vi "SIRDualSlices.vi"(8 "P":cluster{"x":dbl, "y":dbl, "z":dbl}={"x"=1.0, "y"=-5.0, "z"=1.0} {"x" format="%.2f"; "z" format="%.2f"; "y" format="%.2f"}, 9 "Variables":T2={"sound spd (cm/s)"=150000, "time step (s)"=1e-09} {"time step (s)" format="%.2e"}, 11 "strip":cluster{"Radius":dbl, "h":dbl, "a":dbl}={"Radius"=10.0, "h"=3.0, "a"=5.0} {"Radius" format="%.2f"; "a" format="%.2f"; "h" format="%.2f"}) -> (0 "r values":T1 {"r5" format="%.4f"; "r4" format="%.4f"; "r3" format="%.4f"; "r2" format="%.4f"; "r1" format="%.4f"; "r0" format="%.4f"}, 1 "lower":dbl[](graph), 2 "upper":dbl[](graph), 3 "h outer strips":dbl[](graph), 4 "delay out":i32, 5 "cap delay pts":i32, 7 "h cap":dbl[](array[numeric]) format="%.2f")   [LabVIEW 2022 SP3]
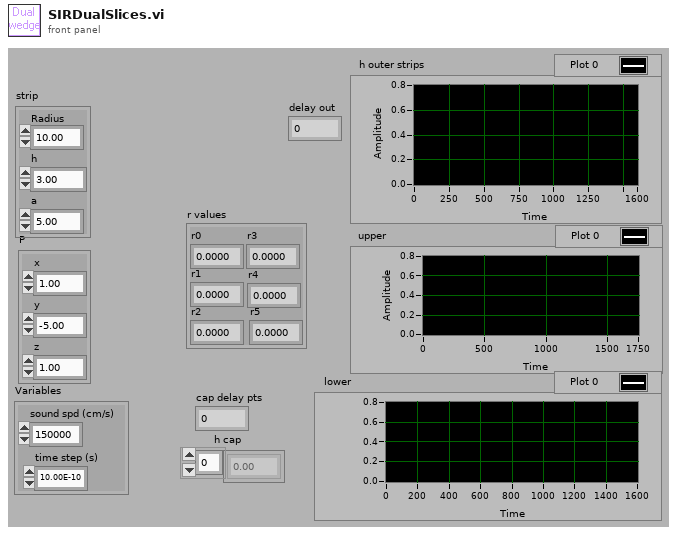
[diagram p1: front panel]
types:
  T1 = cluster{"r0":dbl, "r1":dbl, "r2":dbl, "r3":dbl, "r4":dbl, "r5":dbl}
  T2 = cluster{"sound spd (cm/s)":i32, "time step (s)":sgl}
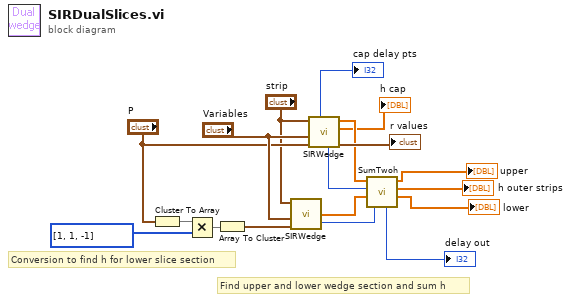
[diagram p0: block diagram]
diagram:
  # "Conversion to find h for lower slice section"
  # "Find upper and lower wedge section and sum h"
  n1 = Cluster To Array(cluster="P") -> (array=w18:dbl[])
  n2 = Multiply(x=w18, y=i32[] [1, 1, -1] ("Array Constant")) -> (x*y=w16:dbl[])
  n3 = Array To Cluster(array=w16) -> (cluster=w10:cluster{"[0]":dbl, "[1]":dbl, "[2]":dbl})
  n4 = call "SIRWedge.vi"("P"=w10, "Variables"="Variables", "strip"="strip") -> ("h wedge"=w6:dbl[], "wedge delay"=w14:i32)  [unwired: 7 out]
  n5 = call "SIRWedge.vi"("P"="P", "Variables"="Variables", "strip"="strip") -> ("r values (cm)"=→"r values":T1, "h cap"=→"h cap":dbl[], "h wedge"=w7:dbl[], "wedge delay"=w13:i32, "cap delay pts"=→"cap delay pts":i32)  [unwired: 4 out]
  n6 = call "SumTwoh.vi"("h1"=w7, "delay1"=w13, "h2"=w6, "delay2"=w14) -> ("delay out"=→"delay out":i32, "upper"=→"upper":dbl[], "h sum"=→"h outer strips":dbl[], "lower"=→"lower":dbl[])  [unwired: 1 out]
